vi "Prog_Status_Handler.vi"(1 "Status Cluster":T2, 3 "Simulate/Run":T1) -> ()   [LabVIEW 2018]
uses:
  Gen Trav/Status_Cluster.ctl
  Gen Trav/Multi_Run_Status.ctl
  Controls/User_Specific_mode.ctl
  Globals/Trav_pos_global.vi
  Globals/Extra_Commands_Global.vi
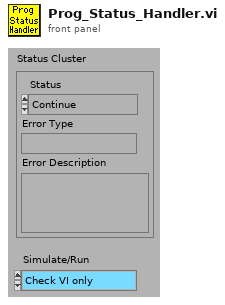
[diagram p1: front panel]
types:
  T1 = typedef "User_Specific_mode.ctl" = enum16{"Check VI only", "Run VI"}
  T2 = typedef "Status_Cluster.ctl" = cluster{"Status":T3, "Error Type":string, "Error Description":string}
  T3 = typedef "Multi_Run_Status.ctl" = enum16{"Continue", "Continue with Error", "Jump to Next Point", "Jump to Next Row", "Jump To Fall Back", "Terminate Run"}
  T4 = typedef "Traverse_cluster.ctl" = cluster{"Start X":sgl, "Start Y":sgl, "Start Z":sgl, "End X":sgl, "End Y":sgl, "End Z":sgl, "No. of pts.":i32, "Spacing":T5, "Filename":path, "Tunnel Speed":dbl, "Averaging time (min)":dbl, "Extra Commands":string, "Carrier_1 Q (l/min)":dbl, "Carrier_2 Q (l/min)":dbl, "Trace Gas Concentration (%)":dbl, "Specific Arguments":string, "Comments":string, "Row No":i32, "Row Type Selector":T6, "Completion time":string, "Row Duration (mins)":dbl, "No. of Valid pts.":i32, "Meas Setup File":string}
  T5 = typedef "Spacing.ctl" = enum16{"Linear", "Log", "Gauss", "Specified", "N/A"}
  T6 = typedef "Multi_run_mode.ctl" = enum16{"Move Traverse Only", "Set Tunnel Speed Only", "Set Source Only", "Set Measurement Conditions", "Single Measurement", "Vertical Profile", "Lateral Profile", "Longitudinal Profile", "Multi-Axis Profile", "Explore Volume", "Auto Calibrate", "Meas Fast FID Bkgnd", "Check Beam Power", "Scanning Valve Measurement", "Run VI Named:", "Set ADAM Ch", "Wait (minutes)", "Send Message", "Synchronize With:", "Fall Back to this Row", "Turn Off Row Repeating", "Traverse 3D Volume", "Blank Row", "Jump to Fall Back Row"}
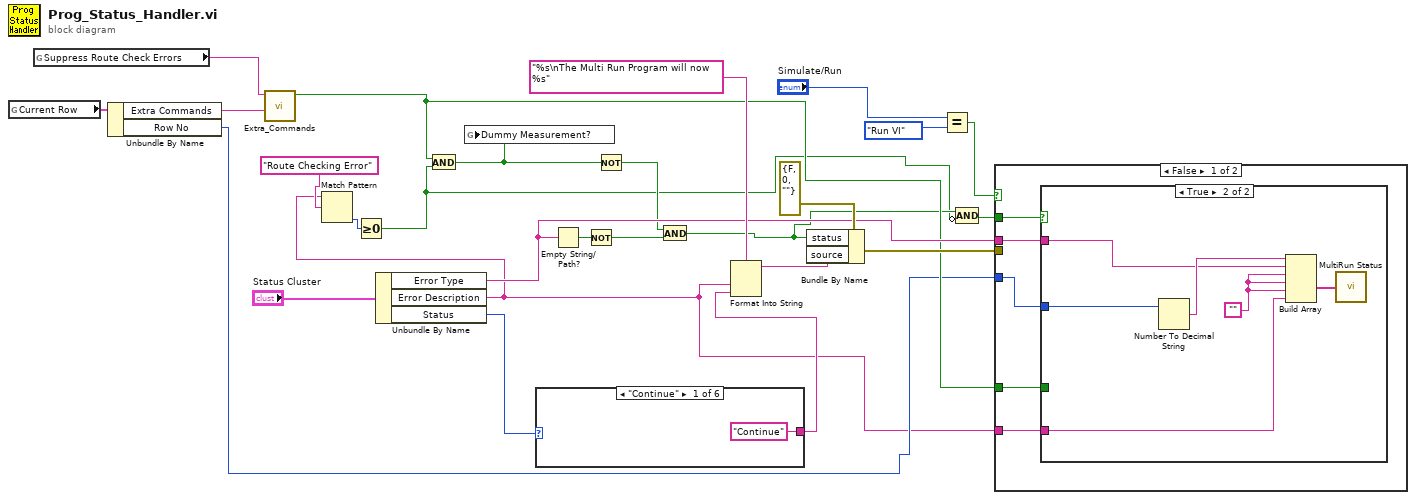
[diagram p0: block diagram]
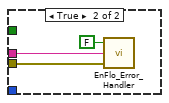
[diagram p3: hidden frame]
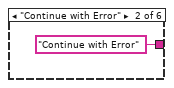
[diagram p4: hidden frame]
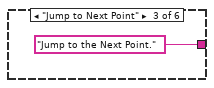
[diagram p5: hidden frame]
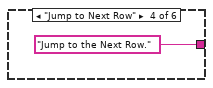
[diagram p6: hidden frame]
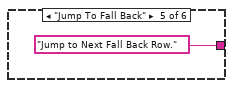
[diagram p7: hidden frame]
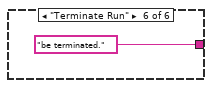
[diagram p8: hidden frame]
diagram:
  n1 = global read "Trav_pos_global.vi" "Current Row"() -> (w8:T4)
  n2 = global read "Extra_Commands_Global.vi" "Suppress Route Check Errors"() -> (w10:string)
  n3 = Unbundle By Name(w8) -> ("Extra Commands"=w9:string, "Row No"=w5:i32)
  n4 = call "Extra_Commands.vi"("String to Search"=w9, "Command"=w10) -> ("Command Found"=w6:bool)  [unwired: 1 in, 4 out]
  n5 = Unbundle By Name("Status Cluster") -> ("Error Type"=w16:string, "Error Description"=w1:string, "Status"=w20:T3)
  n6 = Match Pattern(string=w1, regular expression="Route Checking Error") -> (offset past match=w14:i32)  [unwired: 4 out]
  n7 = Greater Or Equal To 0?(x=w14) -> (x >= 0?=w3:bool)
  n8 = And(x=w6, y=w3) -> (x .and. y?=w11:bool)
  n9 = global write "Trav_pos_global.vi" "Dummy Measurement?"(w11) -> ()
  n10 = case shown="\"Continue\"" w20 {
    tunnel: ["Continue" "Continue with Error" "Jump to the Next Point." "Jump to the Next Row." "Jump to Next Fall Back Row." "be terminated."] -> w26
    frame "Continue" {
    }
    frame "Continue with Error" {
    }
    frame "Jump to Next Point" {
    }
    frame "Jump to Next Row" {
    }
    frame "Jump To Fall Back" {
    }
    frame "Terminate Run" {
    }
  }
  n11 = Empty String/Path?(string/path=w16) -> (empty?=w19:bool)
  n12 = Not(x=w19) -> (.not. x?=w13:bool)
  n13 = Not(x=w11) -> (.not. x?=w12:bool)
  n14 = And(x=w12, y=w13) -> (x .and. y?=w4:bool)
  n15 = Format Into String(format string="%s\nThe Multi Run Program will now %s" ("Format String"), w1, w26) -> (resulting string=w22:string)  [unwired: 2 in, 1 out]
  n16 = Bundle By Name(cluster=errorcluster {"status"=FALSE, "code"=0, "source"=""} ("error in (no error)"), "status"=w4, "source"=w22) -> (w24:errorcluster)
  n17 = Equal?(x="Simulate/Run", y=User_Specific_mode."Run VI" ("Simulate/Run")) -> (x = y?=w7:bool)
  n18 = Compound Arithmetic op=AND(w4, invert w3) -> (w2:bool)
  n19 = case shown="False" w7 {
    tunnel: w24 -> [_ w46]
    tunnel: w16 -> [w35 w45]
    tunnel: w6 -> [w37 _]
    tunnel: w5 -> [w36 _]
    tunnel: w2 -> [w34 _]
    tunnel: w1 -> [w33 _]
    frame False {
      n20 = case shown="True" w34 {
        tunnel: w37 -> [_ _]
        tunnel: w36 -> [_ w42]
        tunnel: w35 -> [_ w40]
        tunnel: w33 -> [_ w39]
        frame False {
        }
        frame True {
          w38 = ""
          n21 = Number To Decimal String(number=w42) -> (decimal integer string=w41:string)  [unwired: 1 in]
          n22 = Build Array(w41, w40, w38, w38, w38, w39) -> (w43:string[])
          n23 = call "MultiRun Status.vi"("Input Array"=w43) -> ()  [unwired: 1 out]
        }
      }
    }
    frame True {
      n24 = call "EnFlo_Error_Handler.vi"("error in (no error)"=w46, "Error Type"=w45, "Dialog Box (T)"=FALSE) -> ()  [unwired: 3 out]
    }
  }
